vi "LaserLineDetection_Intensity_DrawCircle.vi"(4 "Color":u32(colorbox)=16711680, 6 "Radius":i32, 8 "Error In":errorcluster, 9 "Y_center":i32, 10 "X_center":i32, 11 "Image in":T1) -> (0 "Error Out":errorcluster, 3 "Image out":T1)   [LabVIEW 2013]
uses:
  <vilib>/vision/Image Controls.llb/IMAQ Image.ctl
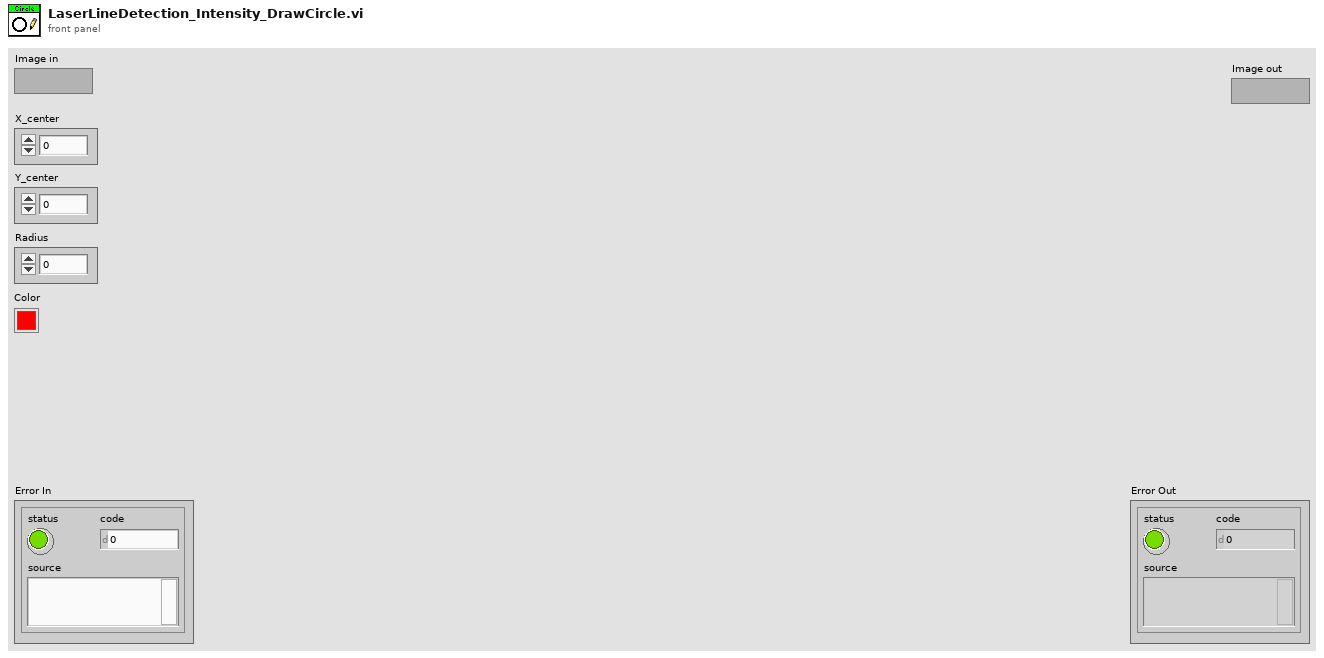
[diagram p1: front panel]
types:
  T1 = typedef "IMAQ Image.ctl" = refnum<image>
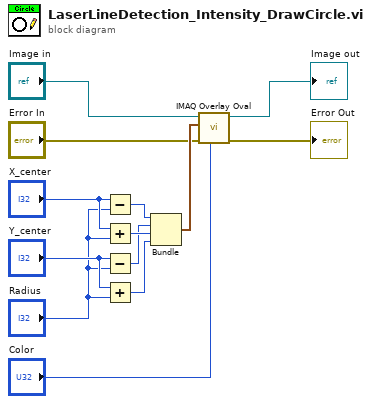
[diagram p0: block diagram]
diagram:
  n1 = Subtract(x="X_center", y="Radius") -> (x-y=w10:i32)
  n2 = Add(x="X_center", y="Radius") -> (x+y=w9:i32)
  n3 = Subtract(x="Y_center", y="Radius") -> (x-y=w6:i32)
  n4 = Add(x="Y_center", y="Radius") -> (x+y=w5:i32)
  n5 = Bundle(w10, w6, w9, w5) -> (w4:cluster{i32, i32, i32, i32})  [unwired: 1 in]
  n6 = call "IMAQ Overlay Oval"("Color"="Color", "error in (no error)"="Error In", "Bounding Rectangle"=w4, "Image"="Image in") -> ("error out"=→"Error Out":errorcluster, "Image Out"=→"Image out":T1)  [unwired: 6 in]
